vi "CRYReplace Signal Type to Channel Name.vi"(10 "Acquisition step in":T1={"Mode"=1, "Name"="", "use ch name"=FALSE, "Record Time"=10.0, "hide rec"=FALSE, "hide play"=FALSE, "rec delay"=0.0, "rec pad"=0.0, "dcc units"=0, "sine gen setting"="", "scope_fft setting"="", "voltmeter setting"="", "rta setting"="", "trig offset(sec)"=0.0, "triggered  record"=FALSE, "trig level"=0.0, "trig unit"=0, "trig slop"=FALSE, "trig timeout(sec)"=0.0, "add record"=FALSE, "EQ"=FALSE, "record table"=[], "play table"=[], "trig channel"="", "Help"=""} {"trig unit" format="%.2f"; "trig level" format="%.2f"; "trig offset(sec)" format="%.2f"; "rec delay" format="%.2f"; "rec pad" format="%.2f"; "Record Time" format="%.2f"}, 11 "Calibration Step in":T2 {"Calibration 2D"."Sens Curve"."Z data" items=["dB", "Lin"]; "Calibration 2D"."Sens Curve"."X data" items=["dB", "Lin"]; "Calibration 2D"."Sens Curve"."Y data" items=["dB", "Lin"]; "Calibration 2D"."Sens Curve"."Z dB ref" format="%.1f"; "Calibration 2D"."Sens Curve"."Z axis" items=["Log", "Lin"]; "Calibration 2D"."Sens Curve"."X dB ref" format="%.1f"; "Calibration 2D"."Sens Curve"."X axis" items=["Log", "Lin"]; "Calibration 2D"."Sens Curve"."Y axis" items=["Log", "Lin"]; "Calibration 2D"."Sens Curve"."Y dB ref" format="%.1f"; "Calibration 2D"."Sens Curve"."Curve"."z" format="%.2f"; "Calibration 2D"."Sens Curve"."Curve"."y" format="%.2f"; "Calibration 2D"."Sens Curve"."Curve"."x" format="%.2f"; "Calibration 2D"."EQ Curve"."Z data" items=["dB", "Lin"]; "Calibration 2D"."EQ Curve"."X data" items=["dB", "Lin"]; "Calibration 2D"."EQ Curve"."Y data" items=["dB", "Lin"]; "Calibration 2D"."EQ Curve"."Z dB ref" format="%.1f"; "Calibration 2D"."EQ Curve"."Z axis" items=["Log", "Lin"]; "Calibration 2D"."EQ Curve"."X dB ref" format="%.1f"; "Calibration 2D"."EQ Curve"."X axis" items=["Log", "Lin"]; "Calibration 2D"."EQ Curve"."Y axis" items=["Log", "Lin"]; "Calibration 2D"."EQ Curve"."Y dB ref" format="%.1f"; "Calibration 2D"."EQ Curve"."Curve"."z" format="%.2f"; "Calibration 2D"."EQ Curve"."Curve"."y" format="%.2f"; "Calibration 2D"."EQ Curve"."Curve"."x" format="%.2f"; "Calibration 2D"."Corr Curve"."Z data" items=["dB", "Lin"]; "Calibration 2D"."Corr Curve"."X data" items=["dB", "Lin"]; "Calibration 2D"."Corr Curve"."Y data" items=["dB", "Lin"]; "Calibration 2D"."Corr Curve"."Z dB ref" format="%.1f"; "Calibration 2D"."Corr Curve"."Z axis" items=["Log", "Lin"]; "Calibration 2D"."Corr Curve"."X dB ref" format="%.1f"; "Calibration 2D"."Corr Curve"."X axis" items=["Log", "Lin"]; "Calibration 2D"."Corr Curve"."Y axis" items=["Log", "Lin"]; "Calibration 2D"."Corr Curve"."Y dB ref" format="%.1f"; "Calibration 2D"."Corr Curve"."Curve"."z" format="%.2f"; "Calibration 2D"."Corr Curve"."Curve"."y" format="%.2f"; "Calibration 2D"."Corr Curve"."Curve"."x" format="%.2f"; "Calibration 2D"."Calibration"."EQ Step size" items=["R10", "R20", "R40", "R80", "User"]; "Calibration 2D"."Calibration"."Corr Step size" items=["R10", "R20", "R40", "R80", "User"]}) -> (0 "Play Signal Type":string[](array[string]), 1 "Play table":string[][](array[string]), 2 "Record Signal Type":string[](array[string]), 3 "record table":string[][](array[string]))   [LabVIEW 2013]
uses:
  Typedef Control/CRYCalibration All Cluster.ctl
  Typedef Control/CRYCalibration 2DCluster.ctl
  Typedef Control/CRYCalibration Cluster.ctl
  Typedef Control/CRYData Cluster.ctl
  Typedef Control/CRYAcquisition Cluster.ctl
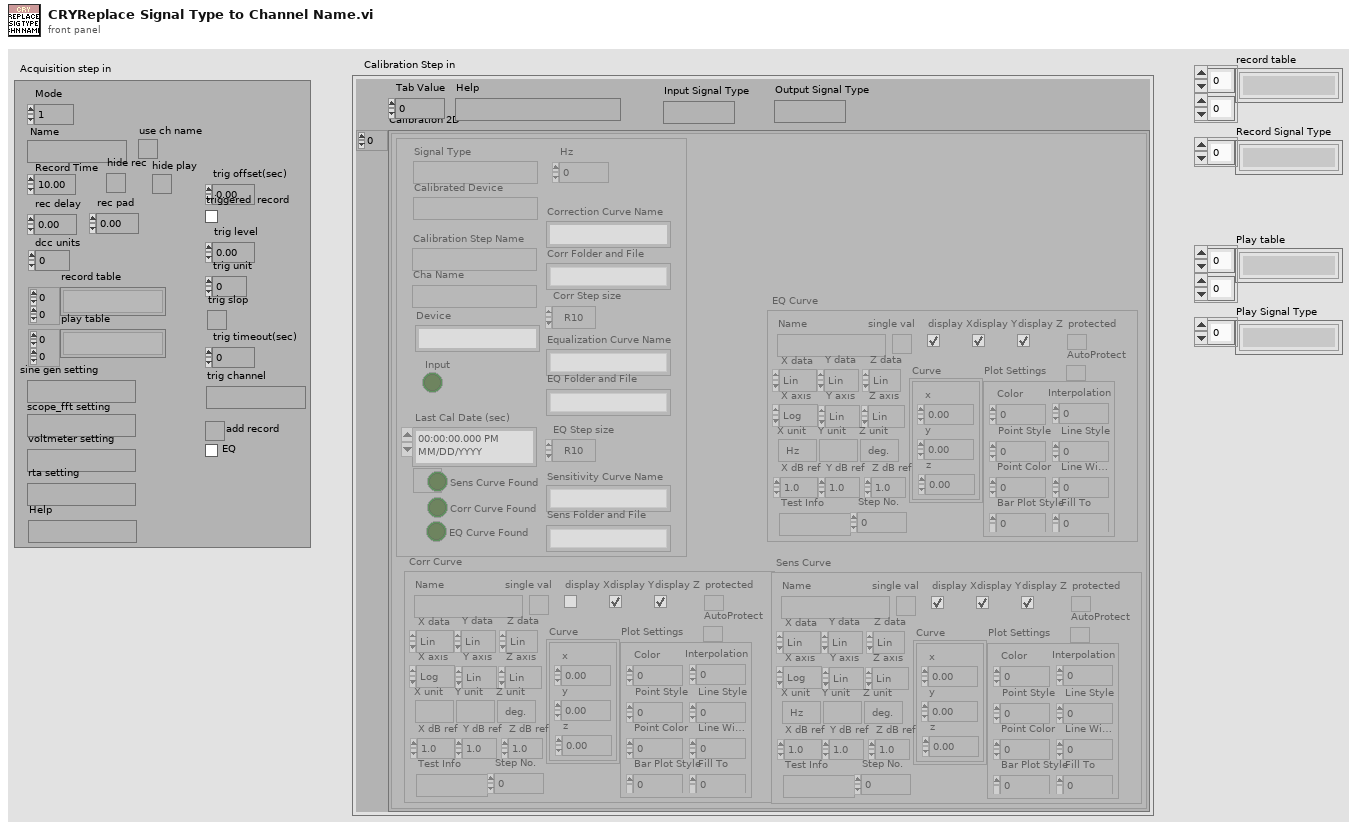
[diagram p1: front panel]
types:
  T1 = typedef "CRYAcquisition Cluster.ctl" = cluster{"Mode":u16, "Name":string, "use ch name":bool, "Record Time":dbl, "hide rec":bool, "hide play":bool, "rec delay":dbl, "rec pad":dbl, "dcc units":i8, "sine gen setting":string, "scope_fft setting":string, "voltmeter setting":string, "rta setting":string, "trig offset(sec)":dbl, "triggered  record":bool, "trig level":dbl, "trig unit":u8, "trig slop":bool, "trig timeout(sec)":dbl, "add record":bool, "EQ":bool, "record table":string[][], "play table":string[][], "trig channel":string, "Help":string}
  T2 = typedef "CRYCalibration All Cluster.ctl" = cluster{"Calibration 2D":T3[], "Help":string, "Tab Value":i32, "Input Signal Type":string, "Output Signal Type":string}
  T3 = typedef "CRYCalibration 2DCluster.ctl" = cluster{"Calibration":T4, "Corr Curve":T5, "EQ Curve":T5, "Sens Curve":T5}
  T4 = typedef "CRYCalibration Cluster.ctl" = cluster{"Calibration Step Name":string, "Device":string, "Correction Curve Name":string, "Equalization Curve Name":string, "Sensitivity Curve Name":string, "Corr Folder and File":string, "EQ Folder and File":string, "Sens Folder and File":string, "Corr Step size":u16, "EQ Step size":u16, "Input":bool, "Last Cal Date (sec)":timestamp, "Cha Name":string, "Corr Curve Found":bool, "EQ Curve Found":bool, "Sens Curve Found":bool, "Signal Type":string, "Calibrated Device":string, "Hz":u32}
  T5 = typedef "CRYData Cluster.ctl" = cluster{"Name":string, "Curve":cluster{"x":dbl, "y":dbl, "z":dbl}[], "X data":u16, "Y data":u16, "Z data":u16, "X axis":u16, "Y axis":u16, "Z axis":u16, "X unit":string, "Y unit":string, "Z unit":string, "X dB ref":dbl, "Y dB ref":dbl, "Z dB ref":dbl, "single val":bool, "protected":bool, "display X":bool, "display Y":bool, "display Z":bool, "Test Info":string, "Step No.":i32, "Plot Settings":cluster{"Color":u32, "Interpolation":u8, "Point Style":u8, "Line Style":u8, "Point Color":u32, "Line Width":u8, "Bar Plot Style":u8, "Fill To":i16}, "AutoProtect":bool}
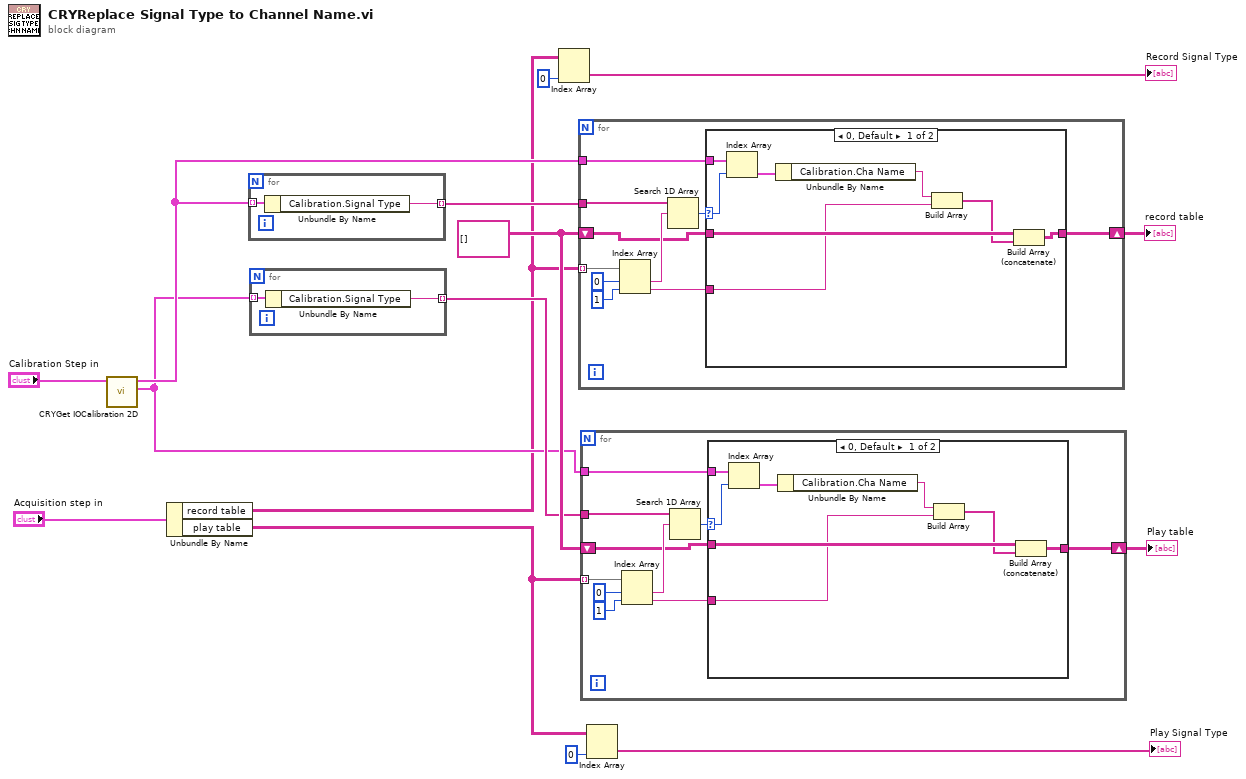
[diagram p0: block diagram]
diagram:
  w11 = string[][] [] ("record table")
  n1 = call "CRYGet IOCalibration 2D.vi"("Calibration"="Calibration Step in") -> ("O_Calibration 2D Out"=w9:T3[], "I_Calibration 2D Out"=w12:T3[])  [unwired: 9 in]
  n2 = Unbundle By Name("Acquisition step in") -> ("record table"=w1:string[][], "play table"=w5:string[][])
  n3 = for {
    tunnel: w12 -> [w17] mode=indexing
    tunnel: [w16] -> w13 mode=indexing
    n4 = Unbundle By Name(w17) -> ("Calibration.Signal Type"=w16:string)
  }
  n5 = for {
    tunnel: w9 -> [w19] mode=indexing
    tunnel: [w18] -> w10 mode=indexing
    n6 = Unbundle By Name(w19) -> ("Calibration.Signal Type"=w18:string)
  }
  n7 = Index Array(array=w1, index (col)=0 ("disabled index (col)")) -> (element=→"Record Signal Type":string[])  [unwired: 1 in]
  n8 = for {
    tunnel: w1 -> [w29] mode=indexing
    tunnel: w13 -> [w26]
    shift-right: [w22] -> w8
    shift-left: w11 -> [w23]
    tunnel: w12 -> [w21]
    n9 = Index Array(array=w29, index #1=0 ("index"), index #2=1 ("index")) -> (element #1=w25:string, element #2=w20:string)
    n10 = Search 1D Array(1D array=w26, element=w25) -> (index of element=w24:i32)  [unwired: 1 in]
    n11 = case shown="0, Default" w24 {
      selector: w24 -> [w35 _]
      tunnel: w23 -> [w37 w38]
      tunnel: [w30 w38] -> w22
      tunnel: w21 -> [w36 _]
      tunnel: w20 -> [w32 _]
      frame 0, Default {
        n12 = Index Array(array=w36, index=w35) -> (element=w34:T3)
        n13 = Unbundle By Name(w34) -> ("Calibration.Cha Name"=w33:string)
        n14 = Build Array(w33, w32) -> (w31:string[])
        n15 = Build Array (concatenate)(w37, w31) -> (w30:string[][])
      }
      frame -1 {
      }
    }
  }
  "record table" <- w8
  n16 = for {
    tunnel: w5 -> [w48] mode=indexing
    tunnel: w10 -> [w45]
    shift-right: [w41] -> w7
    shift-left: w11 -> [w42]
    tunnel: w9 -> [w40]
    n17 = Index Array(array=w48, index #1=0 ("index"), index #2=1 ("index")) -> (element #1=w44:string, element #2=w39:string)
    n18 = Search 1D Array(1D array=w45, element=w44) -> (index of element=w43:i32)  [unwired: 1 in]
    n19 = case shown="0, Default" w43 {
      selector: w43 -> [w54 _]
      tunnel: w42 -> [w56 w57]
      tunnel: [w49 w57] -> w41
      tunnel: w40 -> [w55 _]
      tunnel: w39 -> [w51 _]
      frame 0, Default {
        n20 = Index Array(array=w55, index=w54) -> (element=w53:T3)
        n21 = Unbundle By Name(w53) -> ("Calibration.Cha Name"=w52:string)
        n22 = Build Array(w52, w51) -> (w50:string[])
        n23 = Build Array (concatenate)(w56, w50) -> (w49:string[][])
      }
      frame -1 {
      }
    }
  }
  "Play table" <- w7
  n24 = Index Array(array=w5, index (col)=0 ("disabled index (col)")) -> (element=→"Play Signal Type":string[])  [unwired: 1 in]
